vi "CalculateRobotVelocityAcceleration.vi"(2 "Velocity Y (ft/s)":dbl, 3 "Velocity X (ft/s)":dbl) -> (0 "Velocity Magnitude (ft/s)":dbl, 1 "Velocity Heading (deg)":dbl)   [LabVIEW 2020]
doc: "Calculates the robot's ground velocity as a field relative heading and a magnitude. Robot acceleration measurements can also be performed here by the user."
uses:
  c2341002-2bfb-48f4-9288-ce4646a7db3d.vi
  ff1c0b8b-c98b-4aa7-8b75-1f936d4f23e4.vi
  5d541a37-830b-4907-b671-0e217b9684a2.vi
  83e180a8-8906-4d32-8e94-6535fbb6adc8.vi
  GlobalDrivebase.vi
panel:
  out "Measured Acceleration (ft/s^2)":dbl format="%.1f"
  in  "Reset Acceleration Measurement":bool
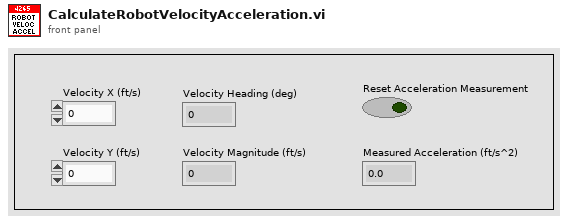
[diagram p1: front panel]
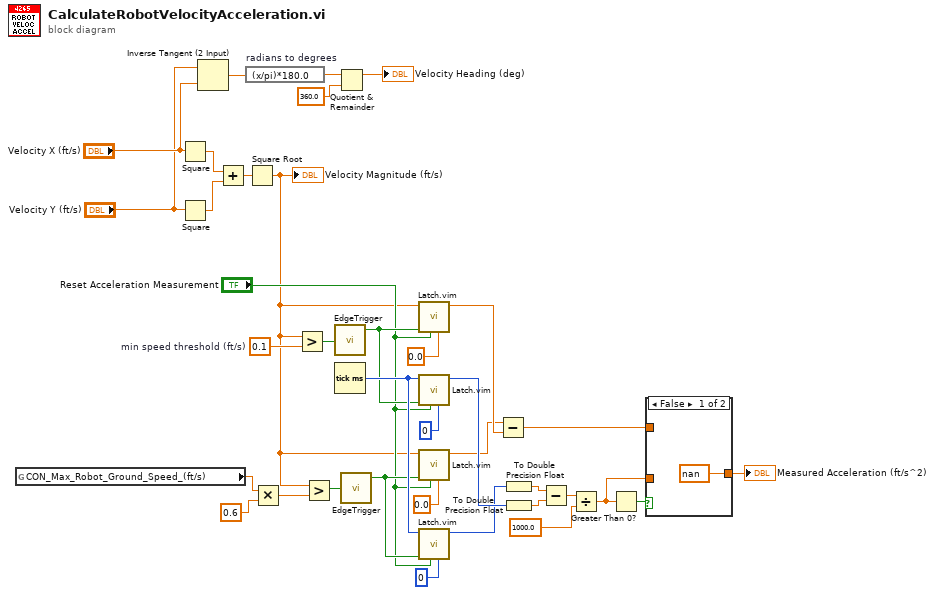
[diagram p0: block diagram]
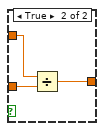
[diagram p2: hidden frame]
diagram:
  w10 = 0.1  # min speed threshold (ft/s)
  n1 = global read "GlobalDrivebase.vi" "CON_Max_Robot_Ground_Speed_(ft/s)"() -> (w7:dbl)
  n2 = Square(x="Velocity X (ft/s)") -> (x^2=w35:dbl)
  n3 = Square(x="Velocity Y (ft/s)") -> (x^2=w36:dbl)
  n4 = Inverse Tangent (2 Input)(1:"Velocity X (ft/s)", 2:"Velocity Y (ft/s)") -> (0:w33:dbl)
  n5 = Add(x=w35, y=w36) -> (x+y=w34:dbl)
  n6 = expression code="(x/pi)*180.0" "radians to degrees"(w33) -> (w31:dbl)
  n7 = Square Root(x=w34) -> (sqrt(x)=w1:dbl)
  "Velocity Magnitude (ft/s)" <- w1
  n8 = Multiply(x=w7, y=0.6) -> (x*y=w5:dbl)
  n9 = Greater?(x=w1, y=w10) -> (0:w9:bool)
  n10 = Greater?(x=w1, y=w5) -> (0:w8:bool)
  n11 = call "EdgeTrigger.vi"("Input Signal"=w9) -> ("Rising Edge Trigger"=w4:bool)  [unwired: 2 out]
  n12 = Tick Count (ms)() -> (millisecond timer value=w16:u32)
  n13 = Quotient & Remainder(x=w31, y=360.0) -> (x-y*floor(x/y)=→"Velocity Heading (deg)":dbl)  [unwired: 1 out]
  n14 = call "EdgeTrigger.vi"("Input Signal"=w8) -> ("Rising Edge Trigger"=w3:bool)  [unwired: 2 out]
  n15 = call "Latch.vim"("Default Value"=0.0, "Reset"="Reset Acceleration Measurement", "Latch Signal"=w4, "Latch Value"=w1) -> ("Latched"=w17:dbl)  [unwired: 7 in]
  n16 = call "Latch.vim"("Default Value"=0, "Reset"="Reset Acceleration Measurement", "Latch Signal"=w4, "Latch Value"=w16) -> ("Latched"=w19:u32)  [unwired: 7 in]
  n17 = call "Latch.vim"("Default Value"=0.0, "Reset"="Reset Acceleration Measurement", "Latch Signal"=w3, "Latch Value"=w1) -> ("Latched"=w13:dbl)  [unwired: 7 in]
  n18 = call "Latch.vim"("Default Value"=0, "Reset"="Reset Acceleration Measurement", "Latch Signal"=w3, "Latch Value"=w16) -> ("Latched"=w18:u32)  [unwired: 7 in]
  n19 = Subtract(x=w13, y=w17) -> (x-y=w26:dbl)
  n20 = To Double Precision Float(number=w18) -> (double precision float=w20:dbl)
  n21 = To Double Precision Float(number=w19) -> (double precision float=w21:dbl)
  n22 = Subtract(x=w20, y=w21) -> (x-y=w22:dbl)
  n23 = Divide(x=w22, y=1000.0) -> (x/y=w25:dbl)
  n24 = Greater Than 0?(x=w25) -> (x > 0?=w24:bool)
  n25 = case shown="False" w24 {
    tunnel: w25 -> [_ w40]
    tunnel: w26 -> [_ w39]
    tunnel: [nan w38] -> w27
    frame False {
    }
    frame True {
      n26 = Divide(x=w39, y=w40) -> (x/y=w38:dbl)
    }
  }
  "Measured Acceleration (ft/s^2)" <- w27
